vi "Heat2D_Solve Y Direction.vi"(5 "Coefficients":T2, 6 "step":i32, 7 "TriDia Cluster":T1, 8 "Boundary Condition":cluster{"type":T3, "Value":dbl[][]}[](array[cluster]) {"type" items=["Dirichlet", "Neumann"]}, 9 "U(n+1/2)":dbl[][](array[numeric])) -> (1 "U(n+1)":dbl[][](array[numeric]))   [LabVIEW 2020, in "NI_PDE.lvlib"]
uses:
  <vilib>/gmath/NI_PDE.lvlib
  <vilib>/gmath/pde.llb/Common/PDE_BC Type.ctl
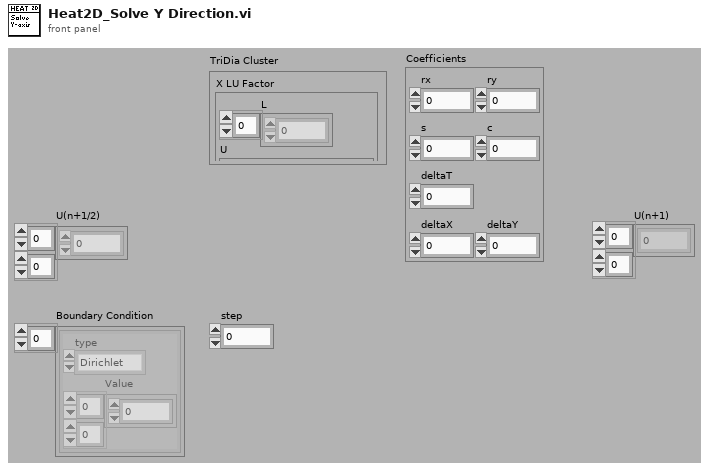
[diagram p1: front panel]
types:
  T1 = cluster{"X LU Factor":cluster{"L":dbl[], "U":cluster{"Diagonal":dbl[], "Super Diagonal":dbl[], "2nd Super Diagonal":dbl[]}, "Pivot":i32[]}, "Y LU Factor":cluster{"L":dbl[], "U":cluster{"Diagonal":dbl[], "Super Diagonal":dbl[], "2nd Super Diagonal":dbl[]}, "Pivot":i32[]}, "X Tridiagonal":cluster{"SubDiagonal":dbl[], "MainDiagonal":dbl[], "SuperDiagonal":dbl[]}, "Y Tridiagonal":cluster{"SubDiagonal":dbl[], "MainDiagonal":dbl[], "SuperDiagonal":dbl[]}}
  T2 = cluster{"rx":dbl, "ry":dbl, "s":dbl, "c":dbl, "deltaT":dbl, "deltaX":dbl, "deltaY":dbl}
  T3 = typedef "NI_PDE.lvlib/PDE_BC Type.ctl" = i32
  T4 = cluster{"L":dbl[], "U":cluster{"Diagonal":dbl[], "Super Diagonal":dbl[], "2nd Super Diagonal":dbl[]}, "Pivot":i32[]}
  T5 = cluster{"SubDiagonal":dbl[], "MainDiagonal":dbl[], "SuperDiagonal":dbl[]}
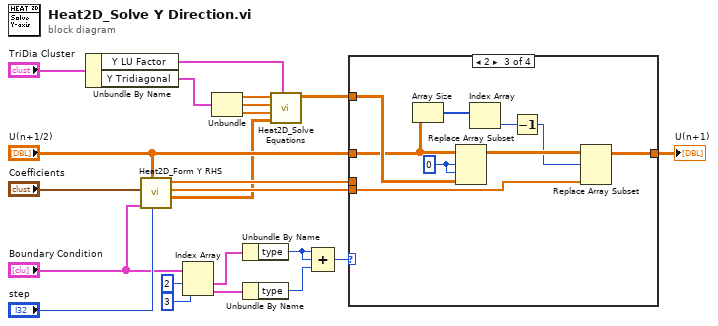
[diagram p0: block diagram]
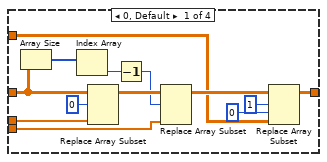
[diagram p2: hidden frame]
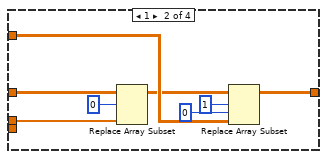
[diagram p3: hidden frame]
diagram:
  n1 = Unbundle By Name("TriDia Cluster") -> ("Y LU Factor"=w7:T4, "Y Tridiagonal"=w6:T5)
  n2 = call <vilib>:"Heat2D_Form Y RHS.vi"("step"="step", "U(n+1/2)"="U(n+1/2)", "Boundary Condition"="Boundary Condition", "Coefficients"="Coefficients") -> ("Y RHS out"=w1:dbl[][], "U down"=w2:dbl[], "U up"=w3:dbl[])  [unwired: 5 out]
  n3 = Index Array(array="Boundary Condition", index #1=2 ("index"), index #2=3 ("index")) -> (element #1=w18:cluster{"type":T3, "Value":dbl[][]}, element #2=w15:cluster{"type":T3, "Value":dbl[][]})
  n4 = Unbundle(w6) -> ("SubDiagonal"=w14:dbl[], "MainDiagonal"=w13:dbl[], "SuperDiagonal"=w12:dbl[])
  n5 = Unbundle By Name(w18) -> ("type"=w16:T3)
  n6 = Unbundle By Name(w15) -> ("type"=w17:T3)
  n7 = call <vilib>:"Heat2D_Solve Equations.vi"("LU Factor"=w7, "RHS"=w1, "SuperDiagonal"=w12, "MainDiagonal"=w13, "SubDiagonal"=w14) -> ("Solution Vector"=w11:dbl[][])  [unwired: 1 in, 5 out]
  n8 = Compound Arithmetic op=ADD(w16, w16, w17) -> (w10:T3)
  n9 = case shown="2" w10 {
    tunnel: w11 -> [w28 w40 w52 w53]
    tunnel: [w26 w38 w47 w53] -> w9
    tunnel: w3 -> [w35 w41 _ _]
    tunnel: w2 -> [w30 _ w46 _]
    tunnel: "U(n+1/2)" -> [w33 w43 w49 _]
    frame 0, Default {
      n10 = Array Size(array=w33) -> (size(s)=w32:i32[])
      n11 = Index Array(array=w32) -> (element=w31:i32)  [unwired: 1 in]
      n12 = Replace Array Subset(array=w33, new element=w35, index (row)=0) -> (w34:dbl[][])  [unwired: 1 in]
      n13 = Decrement(x=w31) -> (x-1=w23:i32)
      n14 = Replace Array Subset(array=w34, new element=w30, index (row)=w23) -> (w29:dbl[][])  [unwired: 1 in]
      n15 = Replace Array Subset(array=w29, new element=w28, index (row)=1, index (col)=0 ("disabled index (col)")) -> (w26:dbl[][])
    }
    frame 1 {
      n16 = Replace Array Subset(array=w43, new element=w41, index (row)=0) -> (w39:dbl[][])  [unwired: 1 in]
      n17 = Replace Array Subset(array=w39, new element=w40, index (row)=1, index (col)=0 ("disabled index (col)")) -> (w38:dbl[][])
    }
    frame 2 {
      w45 = 0 ("index (row)")
      n18 = Array Size(array=w49) -> (size(s)=w48:i32[])
      n19 = Replace Array Subset(array=w49, new element=w52, index (row)=w45, index (col)=w45) -> (w51:dbl[][])
      n20 = Index Array(array=w48) -> (element=w50:i32)  [unwired: 1 in]
      n21 = Decrement(x=w50) -> (x-1=w44:i32)
      n22 = Replace Array Subset(array=w51, new element=w46, index (row)=w44) -> (w47:dbl[][])  [unwired: 1 in]
    }
    frame 3 {
    }
  }
  "U(n+1)" <- w9
